vi "Begin.vi"(8 "error in":errorcluster) -> (0 "error out":errorcluster)   [LabVIEW 2020]
doc: "Called before other user functions, this VI is expected to open initial I/O refnums, load in file data, and do all program initialization. Notice that the <B>error out</B> terminal is simply used for data flow. Wiring it to other structures or subVIs ensures that this VI runs first."
uses:
  <vilib>/Rock Robotics/SystemInterfaces/DIO/FPGA_DIOPWMChannel.ctl
  <vilib>/Rock Robotics/WPI/DriverStation/WPI_DriverStationRobotMode2.ctl
  <vilib>/Rock Robotics/WPI/Joystick/WPI_JoystickDeviceEnum.ctl
  <vilib>/Rock Robotics/WPI/SafetyOutput/WPI_SafetyOutputConfigMenu.ctl
  <vilib>/Rock Robotics/WPI/ThirdParty/Phoenix-LabVIEW/Motor Controller/Controls/CTRE_Phoenix_MotorControl_NeutralMode.ctl
  <vilib>/Rock Robotics/WPI/RobotDrive/WPI_RobotDriveDevRef.ctl
  <vilib>/Rock Robotics/WPI/MotorControl/WPI_MotorControlDeviceRef.ctl
  <vilib>/Rock Robotics/WPI/MotorControl/WPI_MotorControlType.ctl
  <vilib>/Rock Robotics/WPI/PWM/WPI_PWMDeadband.ctl
  <vilib>/Rock Robotics/SystemInterfaces/DIO/FPGA_DIOChannel.ctl
  <vilib>/Rock Robotics/WPI/ThirdParty/Phoenix-LabVIEW/Motor Controller/Controls/CTRE_Phoenix_MotorControl_FeedbackDevice.ctl
  <vilib>/Rock Robotics/SystemInterfaces/AI/FPGA_AIChannel.ctl
  <vilib>/Rock Robotics/WPI/RobotDrive/WPI_RobotDriveOpen2MotorWithTalonSRX.vi
  Robot Global Data.vi
  <vilib>/Rock Robotics/Network Tables/NT Write String Array.vi
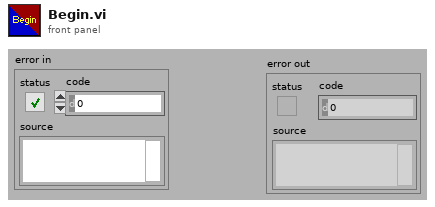
[diagram p1: front panel]
types:
  T1 = typedef "FPGA_AIChannel.ctl" = enum8{"AI 0", "AI 1", "AI 2", "AI 3", "AI MXP 0", "AI MXP 1", "AI MXP 2", "AI MXP 3", "Invalid"}
  T2 = typedef "CTRE_Phoenix_MotorControl_FeedbackDevice.ctl" = i8
  T3 = typedef "CTRE_Phoenix_MotorControl_NeutralMode.ctl" = enum8{"EEPROMSetting", "Override to Coast", "Override to Brake"}
  T4 = typedef "WPI_SafetyOutputConfigMenu.ctl" = enum16{"Enable", "Disable"}
  T5 = typedef "WPI_RobotDriveDevRef.ctl" = cluster{"DevStatus":errorcluster, "Motors[]":T6[], "Square Inputs":bool, "Max Output":dbl}
  T6 = typedef "WPI_MotorControlDeviceRef.ctl" = cluster{"DeviceStatus":errorcluster, "Type":T7, "PWM":cluster{"PWM Channel":T8, "DeadBand":T9}, "CAN":cluster{"Device Number":u8, "SetOutput VI Ref":variant, "GetOutput VI Ref":variant, "Enable VI Ref":variant, "Disable VI Ref":variant, "Data":variant}, "Invert":bool, "DIO PWM":cluster{"PWM \"Enable\" Channel":T8, "DIOChannel":T10, "PWM Rate":dbl}}
  T7 = typedef "WPI_MotorControlType.ctl" = enum16{"PWM", "CAN", "DIO PWM"}
  T8 = typedef "FPGA_DIOPWMChannel.ctl" = enum8{"PWM 0", "PWM 1", "PWM 2", "PWM 3", "PWM 4", "PWM 5", "PWM 6", "PWM 7", "PWM 8", "PWM 9", "PWM MXP 0", "PWM MXP 1", "PWM MXP 2", "PWM MXP 3", "PWM MXP 4", "PWM MXP 5", "PWM MXP 6", "PWM MXP 7", "PWM MXP 8", "PWM MXP 9", "Invalid"}
  T9 = typedef "WPI_PWMDeadband.ctl" = cluster{"Name":string, "maxPositivePwm":i32, "minPositivePwm":i32, "centerPwm":i32, "maxNegativePwm":i32, "minNegativePwm":i32, "angularRange":u16}
  T10 = typedef "FPGA_DIOChannel.ctl" = enum8{"DIO 0", "DIO 1", "DIO 2", "DIO 3", "DIO 4", "DIO 5", "DIO 6", "DIO 7", "DIO 8", "DIO 9", "DIO MXP 0", "DIO MXP 1", "DIO MXP 2", "DIO MXP 3", "DIO MXP 4", "DIO MXP 5", "DIO MXP 6", "DIO MXP 7", "DIO MXP 8", "DIO MXP 9", "DIO MXP 10", "DIO MXP 11", "DIO MXP 12", "DIO MXP 13", "DIO MXP 14", "DIO MXP 15", "SPI Port CS1", "SPI Port CS2", "SPI Port CS3", "SPI Port MISO", "SPI Port MOSI", "Invalid"}
  T11 = typedef "WPI_JoystickDeviceEnum.ctl" = enum16{"USB 0", "USB 1", "USB 2", "USB 3", "USB 4", "USB 5"}
  T12 = typedef "WPI_DriverStationRobotMode2.ctl" = enum16{"Autonomous Disabled", "Autonomous Enabled", "Teleop Disabled", "Teleop Enabled", "Disconnected", "Finish", "Test Disabled", "Test Enabled", "Emergency Stopped"}
  T13 = typedef "WPI_JoystickDevRef.ctl" = cluster{"Device":T11}
  T14 = typedef "WPI_AnalogChannelDevRef.ctl" = cluster{"DevStatus":errorcluster, "Analog Channel":T1}
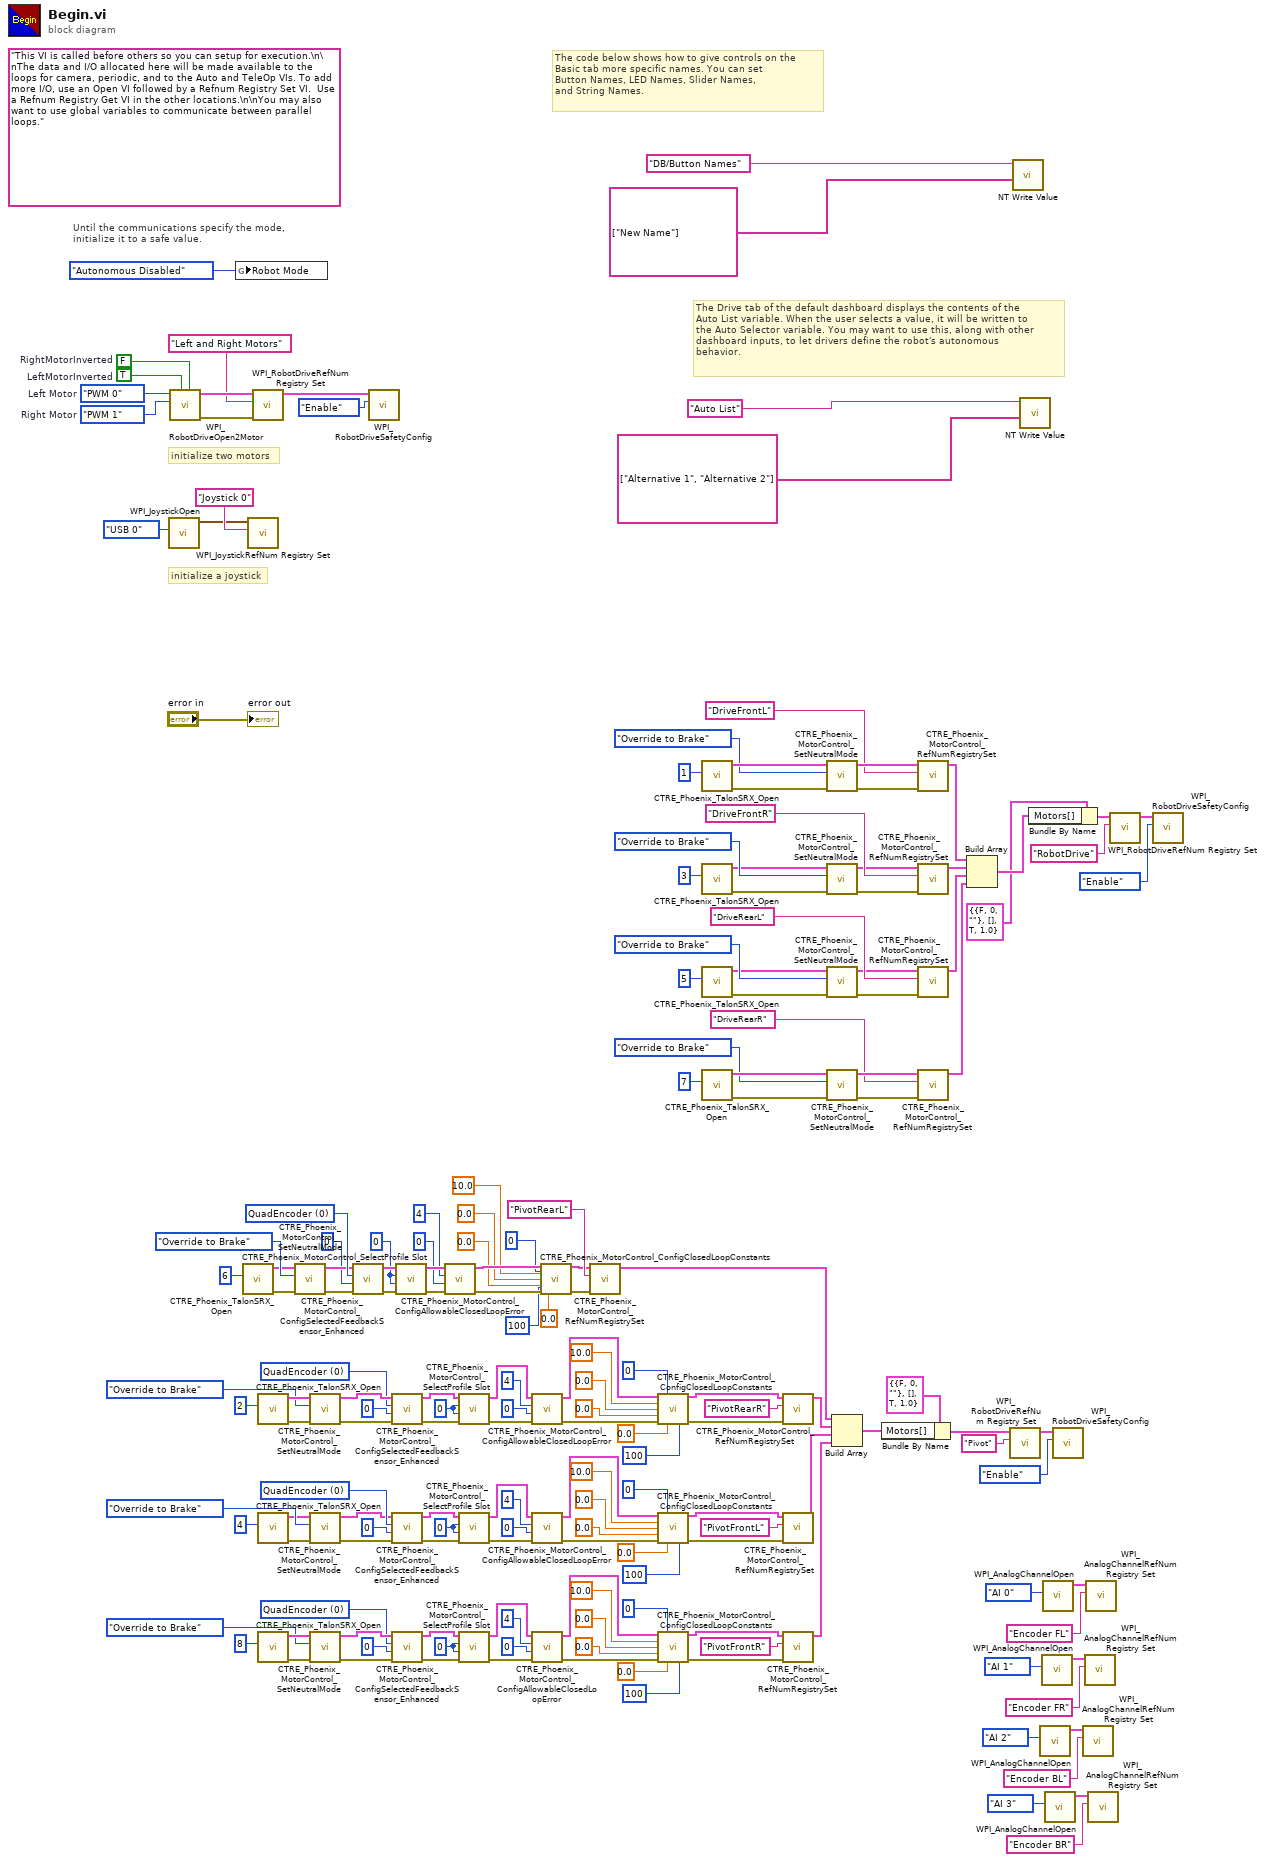
[diagram p0: block diagram]
diagram:
  w29 = 0 ("slotIdx")
  w22 = T2 0 items=["QuadEncoder"=0, "Analog"=2, "Tachometer"=4, "Pulse Width Encoded Position"=8, "Sensor Sum (S0 + S1)"=9, "Sensor Difference (D0 - D1)"=10, "Remote Source 0"=11, "Remote Source 1"=12, "Software Emulated"=15] ("Feedback Device")
  w54 = 0 ("slotIdx")
  w61 = T2 0 items=["QuadEncoder"=0, "Analog"=2, "Tachometer"=4, "Pulse Width Encoded Position"=8, "Sensor Sum (S0 + S1)"=9, "Sensor Difference (D0 - D1)"=10, "Remote Source 0"=11, "Remote Source 1"=12, "Software Emulated"=15] ("Feedback Device")
  w75 = 0 ("slotIdx")
  w68 = T2 0 items=["QuadEncoder"=0, "Analog"=2, "Tachometer"=4, "Pulse Width Encoded Position"=8, "Sensor Sum (S0 + S1)"=9, "Sensor Difference (D0 - D1)"=10, "Remote Source 0"=11, "Remote Source 1"=12, "Software Emulated"=15] ("Feedback Device")
  w102 = 0 ("slotIdx")
  w109 = T2 0 items=["QuadEncoder"=0, "Analog"=2, "Tachometer"=4, "Pulse Width Encoded Position"=8, "Sensor Sum (S0 + S1)"=9, "Sensor Difference (D0 - D1)"=10, "Remote Source 0"=11, "Remote Source 1"=12, "Software Emulated"=15] ("Feedback Device")
  (unwired) "This VI is called before others so you can setup for execution.\n\nThe data and I/O allocated here will be made available to the loops for camera, periodic, and to the Auto and TeleOp VIs. To add more I/O, use an Open VI followed by a Refnum Registry Set VI.  Use a Refnum Registry Get VI in the other locations.\n\nYou may also want to use global variables to communicate between parallel loops."
  w176 = FPGA_DIOPWMChannel."PWM 1"  # Right Motor
  w177 = FPGA_DIOPWMChannel."PWM 0"  # Left Motor
  w181 = TRUE  # LeftMotorInverted
  w182 = FALSE  # RightMotorInverted
  # "The Drive tab of the default dashboard displays the contents of the\nAuto List variable. When the user selects a value, it will be written to\nthe Auto Selector variable. You may want to use this, along with other\ndashboard inputs, to let drivers define the robot's autonomous\nbehavior."
  # "The code below shows how to give controls on the\nBasic tab more specific names. You can set\nButton Names, LED Names, Slider Names,\nand String Names."
  # "initialize a joystick"
  # "Until the communications specify the mode,\ninitialize it to a safe value."
  # "initialize two motors"
  n1 = call <vilib>:"WPI_JoystickOpen.vi"("JoystickDevice"=WPI_JoystickDeviceEnum."USB 0") -> ("JoystickDevRef"=w171:T13)  [unwired: 10 in]
  n2 = call-poly <vilib>:"WPI_RobotDriveOpen2Motor.vi"("Right Motor Inverted"=w182, "Left Motor Inverted"=w181, "Right Motor"=w176, "Left Motor"=w177) -> ("error out"=w178:errorcluster, "RobotDriveDevRef"=w180:T5)  [unwired: 1 in, 5 out]
  n3 = global write "Robot Global Data.vi" "Robot Mode"(WPI_DriverStationRobotMode2."Autonomous Disabled" ("Robot Mode")) -> ()
  n4 = call <vilib>:"CTRE_Phoenix_TalonSRX_Open.vi"("Device Number"=6) -> ("error out"=w106:errorcluster, "PhoenixMotorControlDevRef"=w143:T6)  [unwired: 9 in]
  n5 = call <vilib>:"WPI_JoystickRefNum Registry Set.vi"("refnum name"="Joystick 0", "JoystickDevRef"=w171) -> ()  [unwired: 8 in, 2 out]
  n6 = call <vilib>:"WPI_RobotDriveRefNum Registry Set.vi"("error in (no error)"=w178, "refnum name"="Left and Right Motors", "RobotDriveDevRef"=w180) -> ("RobotDriveDevRef"=w175:T5)  [unwired: 1 in, 7 out]
  n7 = call <vilib>:"CTRE_Phoenix_TalonSRX_Open.vi"("Device Number"=2) -> ("error out"=w71:errorcluster, "PhoenixMotorControlDevRef"=w66:T6)  [unwired: 9 in]
  n8 = call <vilib>:"CTRE_Phoenix_TalonSRX_Open.vi"("Device Number"=4) -> ("error out"=w58:errorcluster, "PhoenixMotorControlDevRef"=w63:T6)  [unwired: 9 in]
  n9 = call <vilib>:"CTRE_Phoenix_TalonSRX_Open.vi"("Device Number"=8) -> ("error out"=w25:errorcluster, "PhoenixMotorControlDevRef"=w20:T6)  [unwired: 9 in]
  n10 = call <vilib>:"CTRE_Phoenix_MotorControl_SetNeutralMode.vi"("error in (no error)"=w106, "Motor Control Neutral Mode"=CTRE_Phoenix_MotorControl_NeutralMode."Override to Brake", "PhoenixMotorControlDevRef"=w143) -> ("error out"=w105:errorcluster, "PhoenixMotorControlDevRef"=w108:T6)  [unwired: 7 in]
  n11 = call <vilib>:"CTRE_Phoenix_MotorControl_SetNeutralMode.vi"("error in (no error)"=w71, "Motor Control Neutral Mode"=CTRE_Phoenix_MotorControl_NeutralMode."Override to Brake", "PhoenixMotorControlDevRef"=w66) -> ("error out"=w72:errorcluster, "PhoenixMotorControlDevRef"=w69:T6)  [unwired: 7 in]
  n12 = call <vilib>:"CTRE_Phoenix_MotorControl_SetNeutralMode.vi"("error in (no error)"=w58, "Motor Control Neutral Mode"=CTRE_Phoenix_MotorControl_NeutralMode."Override to Brake", "PhoenixMotorControlDevRef"=w63) -> ("error out"=w57:errorcluster, "PhoenixMotorControlDevRef"=w60:T6)  [unwired: 7 in]
  n13 = call <vilib>:"CTRE_Phoenix_MotorControl_SetNeutralMode.vi"("error in (no error)"=w25, "Motor Control Neutral Mode"=CTRE_Phoenix_MotorControl_NeutralMode."Override to Brake", "PhoenixMotorControlDevRef"=w20) -> ("error out"=w26:errorcluster, "PhoenixMotorControlDevRef"=w23:T6)  [unwired: 7 in]
  n14 = call <vilib>:"CTRE_Phoenix_MotorControl_ConfigSelectedFeedbackSensor_Enhanced.vi"("error in (no error)"=w105, "pidLoopIdx"=0, "Feedback Device"=w109, "PhoenixMotorControlDevRef"=w108) -> ("error out"=w104:errorcluster, "PhoenixMotorControlDevRef"=w103:T6)  [unwired: 6 in]
  n15 = call <vilib>:"WPI_RobotDriveSafetyConfig.vi"("mode"=WPI_SafetyOutputConfigMenu."Enable", "RobotDriveDevRef"=w175) -> ()  [unwired: 8 in, 2 out]
  n16 = call <vilib>:"CTRE_Phoenix_MotorControl_ConfigSelectedFeedbackSensor_Enhanced.vi"("error in (no error)"=w72, "pidLoopIdx"=0, "Feedback Device"=w68, "PhoenixMotorControlDevRef"=w69) -> ("error out"=w73:errorcluster, "PhoenixMotorControlDevRef"=w74:T6)  [unwired: 6 in]
  n17 = call <vilib>:"CTRE_Phoenix_MotorControl_ConfigSelectedFeedbackSensor_Enhanced.vi"("error in (no error)"=w57, "pidLoopIdx"=0, "Feedback Device"=w61, "PhoenixMotorControlDevRef"=w60) -> ("error out"=w56:errorcluster, "PhoenixMotorControlDevRef"=w55:T6)  [unwired: 6 in]
  n18 = call <vilib>:"CTRE_Phoenix_MotorControl_ConfigSelectedFeedbackSensor_Enhanced.vi"("error in (no error)"=w26, "pidLoopIdx"=0, "Feedback Device"=w22, "PhoenixMotorControlDevRef"=w23) -> ("error out"=w27:errorcluster, "PhoenixMotorControlDevRef"=w28:T6)  [unwired: 6 in]
  n19 = call <vilib>:"CTRE_Phoenix_MotorControl_SelectProfile Slot.vi"("error in (no error)"=w104, "pidLoopIdx"=w102, "slotIdx"=w102, "PhoenixMotorControlDevRef"=w103) -> ("error out"=w101:errorcluster, "PhoenixMotorControlDevRef"=w100:T6)  [unwired: 6 in]
  n20 = call <vilib>:"CTRE_Phoenix_MotorControl_ConfigAllowableClosedLoopError.vi"("error in (no error)"=w101, "slotIdx"=u32 0, "allowableClosedLoopError"=4, "PhoenixMotorControlDevRef"=w100) -> ("error out"=w96:errorcluster, "PhoenixMotorControlDevRef"=w97:T6)  [unwired: 6 in]
  n21 = call <vilib>:"CTRE_Phoenix_MotorControl_SelectProfile Slot.vi"("error in (no error)"=w73, "pidLoopIdx"=w75, "slotIdx"=w75, "PhoenixMotorControlDevRef"=w74) -> ("error out"=w76:errorcluster, "PhoenixMotorControlDevRef"=w77:T6)  [unwired: 6 in]
  n22 = call <vilib>:"CTRE_Phoenix_MotorControl_SelectProfile Slot.vi"("error in (no error)"=w56, "pidLoopIdx"=w54, "slotIdx"=w54, "PhoenixMotorControlDevRef"=w55) -> ("error out"=w53:errorcluster, "PhoenixMotorControlDevRef"=w52:T6)  [unwired: 6 in]
  n23 = call <vilib>:"CTRE_Phoenix_MotorControl_SelectProfile Slot.vi"("error in (no error)"=w27, "pidLoopIdx"=w29, "slotIdx"=w29, "PhoenixMotorControlDevRef"=w28) -> ("error out"=w30:errorcluster, "PhoenixMotorControlDevRef"=w31:T6)  [unwired: 6 in]
  n24 = call <vilib>:"CTRE_Phoenix_MotorControl_ConfigAllowableClosedLoopError.vi"("error in (no error)"=w76, "slotIdx"=u32 0, "allowableClosedLoopError"=4, "PhoenixMotorControlDevRef"=w77) -> ("error out"=w81:errorcluster, "PhoenixMotorControlDevRef"=w80:T6)  [unwired: 6 in]
  n25 = call <vilib>:"CTRE_Phoenix_MotorControl_ConfigAllowableClosedLoopError.vi"("error in (no error)"=w53, "slotIdx"=u32 0, "allowableClosedLoopError"=4, "PhoenixMotorControlDevRef"=w52) -> ("error out"=w48:errorcluster, "PhoenixMotorControlDevRef"=w49:T6)  [unwired: 6 in]
  n26 = call <vilib>:"CTRE_Phoenix_MotorControl_ConfigAllowableClosedLoopError.vi"("error in (no error)"=w30, "slotIdx"=u32 0, "allowableClosedLoopError"=4, "PhoenixMotorControlDevRef"=w31) -> ("error out"=w35:errorcluster, "PhoenixMotorControlDevRef"=w34:T6)  [unwired: 6 in]
  n27 = call <vilib>:"CTRE_Phoenix_MotorControl_ConfigClosedLoopConstants.vi"("PhoenixMotorControlDevRef"=w97, "slotIdx"=0, "P"=10.0, "I"=0.0, "D"=0.0, "error in (no error)"=w96, "F"=0.0, "timeoutMs"=100) -> ("PhoenixMotorControlDevRef"=w89:T6, "error out"=w88:errorcluster)  [unwired: 6 in]
  n28 = call <vilib>:"CTRE_Phoenix_MotorControl_RefNumRegistrySet.vi"("error in (no error)"=w88, "refnum name"="PivotRearL", "PhoenixMotorControlDevRef"=w89) -> ("PhoenixMotorControlDevRef"=w149:T6)  [unwired: 7 in, 1 out]
  n29 = call <vilib>:"CTRE_Phoenix_MotorControl_ConfigClosedLoopConstants.vi"("PhoenixMotorControlDevRef"=w80, "slotIdx"=0, "P"=10.0, "I"=0.0, "D"=0.0, "error in (no error)"=w81, "F"=0.0, "timeoutMs"=100) -> ("PhoenixMotorControlDevRef"=w13:T6, "error out"=w14:errorcluster)  [unwired: 6 in]
  n30 = call <vilib>:"CTRE_Phoenix_MotorControl_ConfigClosedLoopConstants.vi"("PhoenixMotorControlDevRef"=w49, "slotIdx"=0, "P"=10.0, "I"=0.0, "D"=0.0, "error in (no error)"=w48, "F"=0.0, "timeoutMs"=100) -> ("PhoenixMotorControlDevRef"=w16:T6, "error out"=w15:errorcluster)  [unwired: 6 in]
  n31 = call <vilib>:"CTRE_Phoenix_MotorControl_ConfigClosedLoopConstants.vi"("PhoenixMotorControlDevRef"=w34, "slotIdx"=0, "P"=10.0, "I"=0.0, "D"=0.0, "error in (no error)"=w35, "F"=0.0, "timeoutMs"=100) -> ("PhoenixMotorControlDevRef"=w18:T6, "error out"=w17:errorcluster)  [unwired: 6 in]
  n32 = call <vilib>:"CTRE_Phoenix_TalonSRX_Open.vi"("Device Number"=1) -> ("error out"=w161:errorcluster, "PhoenixMotorControlDevRef"=w160:T6)  [unwired: 9 in]
  n33 = call <vilib>:"CTRE_Phoenix_TalonSRX_Open.vi"("Device Number"=3) -> ("error out"=w136:errorcluster, "PhoenixMotorControlDevRef"=w137:T6)  [unwired: 9 in]
  n34 = call <vilib>:"CTRE_Phoenix_TalonSRX_Open.vi"("Device Number"=5) -> ("error out"=w122:errorcluster, "PhoenixMotorControlDevRef"=w123:T6)  [unwired: 9 in]
  n35 = call <vilib>:"CTRE_Phoenix_TalonSRX_Open.vi"("Device Number"=7) -> ("error out"=w129:errorcluster, "PhoenixMotorControlDevRef"=w128:T6)  [unwired: 9 in]
  n36 = call <vilib>:"CTRE_Phoenix_MotorControl_RefNumRegistrySet.vi"("error in (no error)"=w14, "refnum name"="PivotRearR", "PhoenixMotorControlDevRef"=w13) -> ("PhoenixMotorControlDevRef"=w112:T6)  [unwired: 7 in, 1 out]
  n37 = call <vilib>:"CTRE_Phoenix_MotorControl_RefNumRegistrySet.vi"("error in (no error)"=w15, "refnum name"="PivotFrontL", "PhoenixMotorControlDevRef"=w16) -> ("PhoenixMotorControlDevRef"=w111:T6)  [unwired: 7 in, 1 out]
  n38 = call <vilib>:"CTRE_Phoenix_MotorControl_RefNumRegistrySet.vi"("error in (no error)"=w17, "refnum name"="PivotFrontR", "PhoenixMotorControlDevRef"=w18) -> ("PhoenixMotorControlDevRef"=w110:T6)  [unwired: 7 in, 1 out]
  n39 = call <vilib>:"CTRE_Phoenix_MotorControl_SetNeutralMode.vi"("error in (no error)"=w161, "Motor Control Neutral Mode"=CTRE_Phoenix_MotorControl_NeutralMode."Override to Brake", "PhoenixMotorControlDevRef"=w160) -> ("error out"=w163:errorcluster, "PhoenixMotorControlDevRef"=w162:T6)  [unwired: 7 in]
  n40 = call <vilib>:"CTRE_Phoenix_MotorControl_SetNeutralMode.vi"("error in (no error)"=w136, "Motor Control Neutral Mode"=CTRE_Phoenix_MotorControl_NeutralMode."Override to Brake", "PhoenixMotorControlDevRef"=w137) -> ("error out"=w134:errorcluster, "PhoenixMotorControlDevRef"=w135:T6)  [unwired: 7 in]
  n41 = call <vilib>:"CTRE_Phoenix_MotorControl_SetNeutralMode.vi"("error in (no error)"=w122, "Motor Control Neutral Mode"=CTRE_Phoenix_MotorControl_NeutralMode."Override to Brake", "PhoenixMotorControlDevRef"=w123) -> ("error out"=w120:errorcluster, "PhoenixMotorControlDevRef"=w121:T6)  [unwired: 7 in]
  n42 = call <vilib>:"CTRE_Phoenix_MotorControl_SetNeutralMode.vi"("error in (no error)"=w129, "Motor Control Neutral Mode"=CTRE_Phoenix_MotorControl_NeutralMode."Override to Brake", "PhoenixMotorControlDevRef"=w128) -> ("error out"=w131:errorcluster, "PhoenixMotorControlDevRef"=w130:T6)  [unwired: 7 in]
  n43 = Build Array(w149, w112, w111, w110) -> (w150:T6[])
  n44 = Bundle By Name(cluster=T5 {"DevStatus"={"status"=FALSE, "code"=0, "source"=""}, "Motors[]"=[], "Square Inputs"=TRUE, "Max Output"=1.0} ("RobotDriveDevRef"), "Motors[]"=w150) -> (w147:T5)
  n45 = call <vilib>:"CTRE_Phoenix_MotorControl_RefNumRegistrySet.vi"("error in (no error)"=w163, "refnum name"="DriveFrontL", "PhoenixMotorControlDevRef"=w162) -> ("PhoenixMotorControlDevRef"=w156:T6)  [unwired: 7 in, 1 out]
  n46 = call <vilib>:"CTRE_Phoenix_MotorControl_RefNumRegistrySet.vi"("error in (no error)"=w134, "refnum name"="DriveFrontR", "PhoenixMotorControlDevRef"=w135) -> ("PhoenixMotorControlDevRef"=w115:T6)  [unwired: 7 in, 1 out]
  n47 = call <vilib>:"CTRE_Phoenix_MotorControl_RefNumRegistrySet.vi"("error in (no error)"=w120, "refnum name"="DriveRearL", "PhoenixMotorControlDevRef"=w121) -> ("PhoenixMotorControlDevRef"=w114:T6)  [unwired: 7 in, 1 out]
  n48 = call <vilib>:"CTRE_Phoenix_MotorControl_RefNumRegistrySet.vi"("error in (no error)"=w131, "refnum name"="DriveRearR", "PhoenixMotorControlDevRef"=w130) -> ("PhoenixMotorControlDevRef"=w113:T6)  [unwired: 7 in, 1 out]
  n49 = Build Array(w156, w115, w114, w113) -> (w155:T6[])
  n50 = call <vilib>:"WPI_RobotDriveRefNum Registry Set.vi"("refnum name"="Pivot", "RobotDriveDevRef"=w147) -> ("RobotDriveDevRef"=w151:T5)  [unwired: 8 in, 1 out]
  n51 = call-poly <vilib>:"NT Write Value.vi"("String Array"=string[] ["New Name"], "Name"="DB/Button Names") -> ()  [unwired: 9 in, 1 out]
  n52 = call-poly <vilib>:"NT Write Value.vi"("String Array"=string[] ["Alternative 1", "Alternative 2"], "Name"="Auto List") -> ()  [unwired: 9 in, 1 out]
  n53 = Bundle By Name(cluster=T5 {"DevStatus"={"status"=FALSE, "code"=0, "source"=""}, "Motors[]"=[], "Square Inputs"=TRUE, "Max Output"=1.0} ("RobotDriveDevRef"), "Motors[]"=w155) -> (w140:T5)
  n54 = call <vilib>:"WPI_AnalogChannelOpen.vi"("Analog Channel"=FPGA_AIChannel."AI 2") -> ("AIDeviceRef"=w7:T14)  [unwired: 9 in, 1 out]
  n55 = call <vilib>:"WPI_AnalogChannelOpen.vi"("Analog Channel"=FPGA_AIChannel."AI 1") -> ("AIDeviceRef"=w4:T14)  [unwired: 9 in, 1 out]
  n56 = call <vilib>:"WPI_AnalogChannelOpen.vi"("Analog Channel"=FPGA_AIChannel."AI 0") -> ("AIDeviceRef"=w2:T14)  [unwired: 9 in, 1 out]
  n57 = call <vilib>:"WPI_AnalogChannelOpen.vi"("Analog Channel"=FPGA_AIChannel."AI 3") -> ("AIDeviceRef"=w8:T14)  [unwired: 9 in, 1 out]
  n58 = call <vilib>:"WPI_RobotDriveSafetyConfig.vi"("mode"=WPI_SafetyOutputConfigMenu."Enable", "RobotDriveDevRef"=w151) -> ()  [unwired: 8 in, 2 out]
  n59 = call <vilib>:"WPI_AnalogChannelRefNum Registry Set.vi"("refnum name"="Encoder BL", "AIDeviceRef"=w7) -> ()  [unwired: 8 in, 2 out]
  n60 = call <vilib>:"WPI_AnalogChannelRefNum Registry Set.vi"("refnum name"="Encoder FR", "AIDeviceRef"=w4) -> ()  [unwired: 8 in, 2 out]
  n61 = call <vilib>:"WPI_AnalogChannelRefNum Registry Set.vi"("refnum name"="Encoder FL", "AIDeviceRef"=w2) -> ()  [unwired: 8 in, 2 out]
  n62 = call <vilib>:"WPI_AnalogChannelRefNum Registry Set.vi"("refnum name"="Encoder BR", "AIDeviceRef"=w8) -> ()  [unwired: 8 in, 2 out]
  n63 = call <vilib>:"WPI_RobotDriveRefNum Registry Set.vi"("refnum name"="RobotDrive", "RobotDriveDevRef"=w140) -> ("RobotDriveDevRef"=w154:T5)  [unwired: 8 in, 1 out]
  n64 = call <vilib>:"WPI_RobotDriveSafetyConfig.vi"("mode"=WPI_SafetyOutputConfigMenu."Enable", "RobotDriveDevRef"=w154) -> ()  [unwired: 8 in, 2 out]
  "error out" <- "error in"
